vi "Menu - Get the 2nd Order Tags__SubVIs-某型振动实验台测试系统.vi"(8 "error in (no error)":errorcluster, 11 "menu in":refnum<k9>) -> (0 "error out":errorcluster, 2 "menu 2nd order tags":string[](array[string]), 3 "menu out":refnum<k9>)   [LabVIEW 2011]
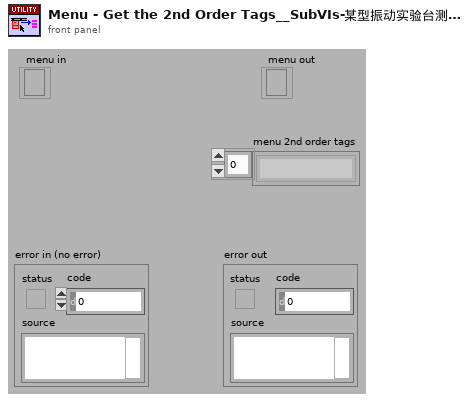
[diagram p1: front panel]
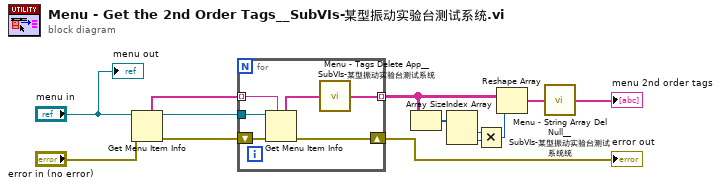
[diagram p0: block diagram]
diagram:
  n1 = Get Menu Item Info(8:"error in (no error)", 11:"menu in") -> (0:w4:errorcluster, 3:w6:refnum<k9>, 5:w5:string[])  [unwired: 5 out]
  n2 = for {
    tunnel: w5 -> [w18] mode=indexing
    tunnel: w6 -> [w19]
    tunnel: [w16] -> w7 mode=indexing
    shift-right: [w14] -> w2
    shift-left: w4 -> [w15]
    n3 = Get Menu Item Info(7:w18, 8:w15, 11:w19) -> (0:w14:errorcluster, 5:w17:string[])  [unwired: 5 out]
    n4 = call "Menu - Tags Delete App__SubVIs-某型振动实验台测试系统.vi"("menu tags in"=w17) -> ("menu tags out"=w16:string[])
  }
  "error out" <- w2
  n5 = Array Size(array=w7) -> (size(s)=w8:i32[])
  n6 = Index Array(array=w8) -> (element #1=w9:i32, element #2=w10:i32)  [unwired: 2 in]
  n7 = Multiply(x=w9, y=w10) -> (x*y=w11:i32)
  n8 = Reshape Array(w7, w11) -> (w12:string[])
  n9 = call "Menu - String Array Del Null__SubVIs-某型振动实验台测试系统统.vi"("Array"=w12) -> ("Out"=→"menu 2nd order tags":string[])
  "menu out" <- "menu in"
